vi "2401 Compliance.vi"(7 "I/V":bool, 9 "Compliance":dbl) -> ()   [LabVIEW 2009]
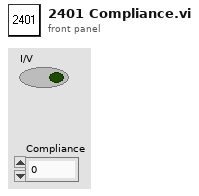
[diagram p1: front panel]
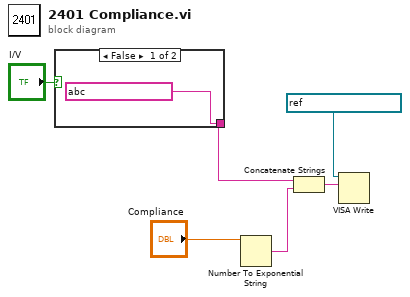
[diagram p0: block diagram]
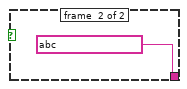
[diagram p2: hidden frame]
diagram:
  n1 = case shown="False" "I/V" {
    tunnel: [string ? ("write buffer") string ? ("write buffer")] -> w5
    frame #0 {
    }
    frame #1 {
    }
  }
  n2 = Number To Exponential String(number="Compliance") -> (E-format string=w3:string)  [unwired: 3 in]
  n3 = Concatenate Strings(w5, w3) -> (w4:string)
  n4 = VISA Write(VISA resource name=refnum<visa-resource-name> ?, write buffer=w4) -> ()  [unwired: 1 in, 3 out]
